vi "Read SP.vi"(8 "error in (no error)":errorcluster, 11 "Change Setpoint MSG in":refnum<class "Change Setpoint MSG.lvclass">) -> (0 "error out":errorcluster, 2 "SP":dbl, 3 "Change Setpoint MSG out":refnum<class "Change Setpoint MSG.lvclass">)   [LabVIEW 2015, in "Alicat Lib.lvlib" / "Change Setpoint MSG.lvclass"]
uses:
  Change Setpoint MSG.lvclass
  Change Setpoint MSG.lvclass/Change Setpoint MSG.ctl
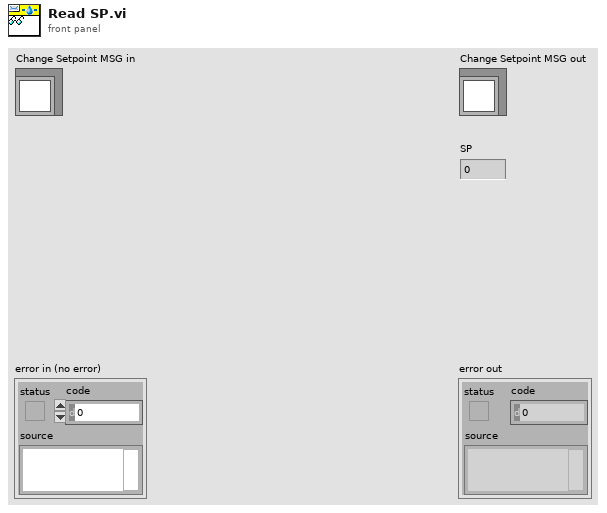
[diagram p1: front panel]
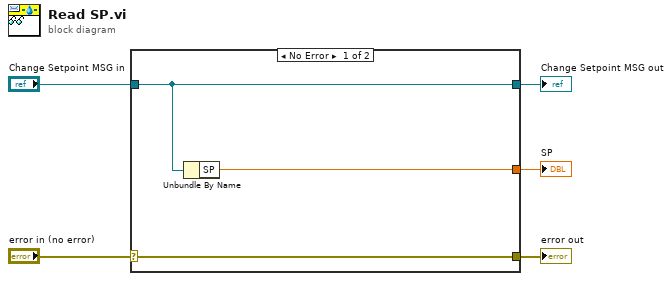
[diagram p0: block diagram]
diagram:
  n1 = case shown="No Error" "error in (no error)" {
    selector: "error in (no error)" -> [w8 w9]
    tunnel: [w8 w9] -> w4
    tunnel: [w7 w10] -> w2
    tunnel: "Change Setpoint MSG in" -> [w7 w10]
    tunnel: [w6 _] -> w1
    frame No Error {
      n2 = Unbundle By Name(w7) -> ("SP"=w6:dbl)
    }
    frame Error {
    }
  }
  "error out" <- w4
  "Change Setpoint MSG out" <- w2
  "SP" <- w1
